vi "RefreshEntireTreeWithGlyphManager.vi"(7 "calling VI in":refnum<vi>, 8 "error in":errorcluster, 9 "glyph manager":T1, 10 "array":T3[](array[typedef]), 11 "tree ref in":refnum<vi>) -> (0 "error out":errorcluster, 1 "glyph manager out":T1)   [LabVIEW 2013, in "NISE_CEF_TreeControl.lvlib"]
doc: "This VI refreshes the complete tree based on the node summary"
uses:
  NISE_CEF_TreeControl.lvlib
  Node/Summary.ctl
  glyph manager/glyph manager.ctl
  <vilib>/picture/picture.llb/imagedata.ctl
  glyph manager/glyph manager.lvlib
  Node/NISE_CEF_Node.lvclass
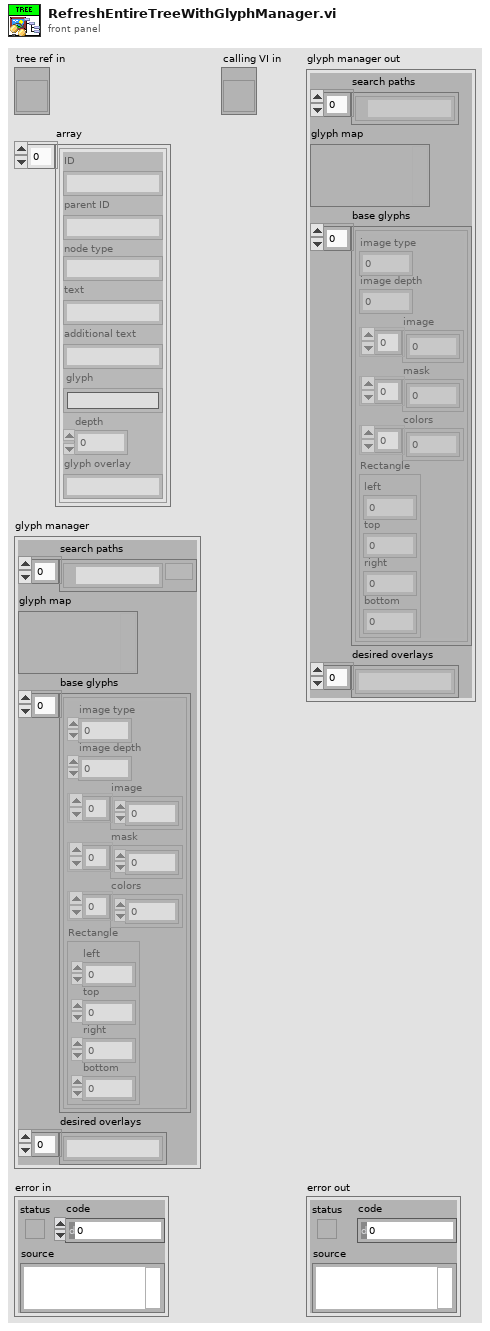
[diagram p1: front panel]
types:
  T1 = typedef "glyph manager.lvlib/glyph manager.ctl" = cluster{"search paths":path[], "glyph map":variant, "base glyphs":T2[], "desired overlays":string[]}
  T2 = typedef "imagedata.ctl" = cluster{"image type":i32, "image depth":i32, "image":u8[], "mask":u8[], "colors":u32[], "Rectangle":cluster{"left":i16, "top":i16, "right":i16, "bottom":i16}}
  T3 = typedef "NISE_CEF_Node.lvclass/Summary.ctl" = cluster{"ID":string, "parent ID":string, "node type":string, "text":string, "additional text":string, "glyph":string, "depth":i32, "glyph overlay":string}
  T4 = cluster{"Left Cell String":string, "Child text":string[], "Child Tag":string, "Item Indent":i32, "Child Only?":bool, "glyph Index":i32}
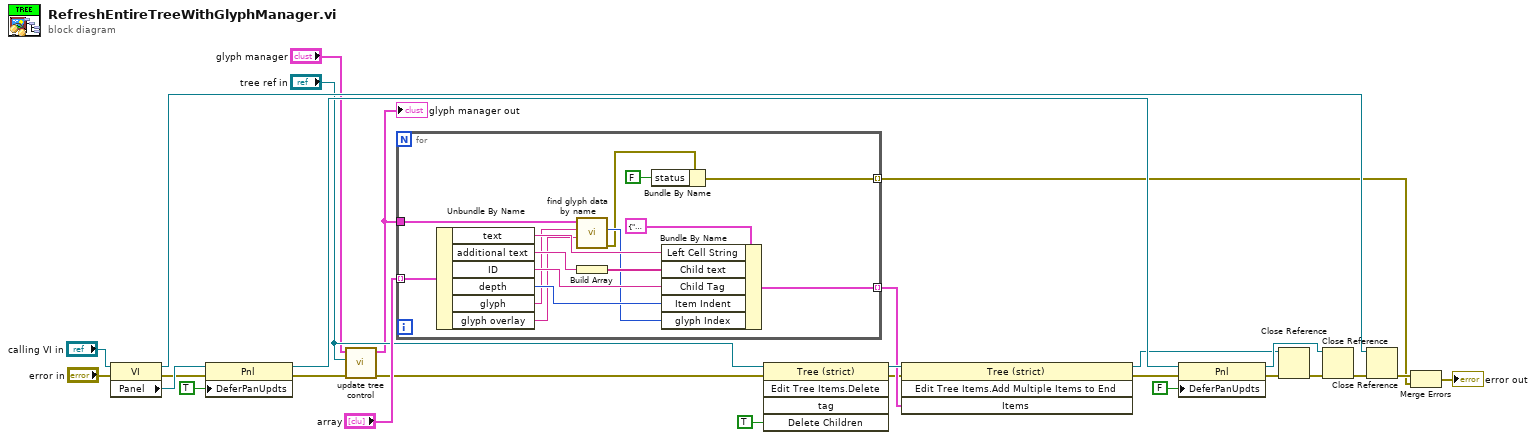
[diagram p0: block diagram]
diagram:
  n1 = property class="VI"(reference="calling VI in", error in="error in") -> (reference out=w17:refnum<vi>, error out=w25:errorcluster, "Panel"=w26:refnum<vi>)
  n2 = property class="Pnl"(reference=w26, error in=w25, "DeferPanUpdts"=TRUE ("Defer Panel Updates")) -> (reference out=w21:refnum<vi>, error out=w11:errorcluster)
  n3 = call "update tree control.vi"("error in"=w11, "tree reference"="tree ref in", "glyph manager in"="glyph manager") -> ("error out"=w5:errorcluster, "glyph manager out"=w1:T1)  [unwired: 7 in]
  "glyph manager out" <- w1
  n4 = for {
    tunnel: "array" -> [w42] mode=indexing
    tunnel: [w40] -> w10 mode=indexing
    tunnel: [w32] -> w2 mode=indexing
    tunnel: w1 -> [w30]
    n5 = Unbundle By Name(w42) -> ("text"=w39:string, "additional text"=w37:string, "ID"=w36:string, "depth"=w35:i32, "glyph"=w29:string, "glyph overlay"=w28:string)
    n6 = call "find glyph data by name.vi"("overlay"=w28, "name"=w29, "glyph manager in"=w30) -> ("error out"=w33:errorcluster, "symbol index"=w34:i32)  [unwired: 5 in, 2 out]
    n7 = Build Array(w37) -> (w38:string[])
    n8 = Bundle By Name(cluster=w33, "status"=FALSE) -> (w32:errorcluster)
    n9 = Bundle By Name(cluster=T4 {"Left Cell String"="", "Child text"=[], "Child Tag"="", "Item Indent"=0, "Child Only?"=FALSE, "glyph Index"=0} ("Item"), "Left Cell String"=w39, "Child text"=w38, "Child Tag"=w36, "Item Indent"=w35, "glyph Index"=w34) -> (w40:T4)
  }
  n10 = invoke class="Tree (strict)" method="Edit Tree Items.Delete"(reference="tree ref in", error in=w5, "Delete Children"=TRUE ("Delete Children?")) -> (reference out=w13:refnum<vi>, error out=w9:errorcluster)  [unwired: 2 in, 3 out]
  n11 = invoke class="Tree (strict)" method="Edit Tree Items.Add Multiple Items to End"(reference=w13, error in=w9, "Items"=w10) -> (reference out=w12:refnum<vi>, error out=w8:errorcluster)  [unwired: 1 in, 2 out]
  n12 = property class="Pnl"(reference=w21, error in=w8, "DeferPanUpdts"=FALSE ("Defer Panel Updates")) -> (reference out=w18:refnum<vi>, error out=w20:errorcluster)
  n13 = Close Reference(reference=w12, error in (no error)=w20) -> (error out=w19:errorcluster)
  n14 = Close Reference(reference=w18, error in (no error)=w19) -> (error out=w16:errorcluster)
  n15 = Close Reference(reference=w17, error in (no error)=w16) -> (error out=w6:errorcluster)
  n16 = Merge Errors(w6, w2) -> (→"error out":errorcluster)
